vi "DAQNavi Read (Analog Wfm 1Chan NSamp).vi"(8 "error in (no error)":errorcluster, 9 "number of samples per channel to read":u32=1000, 10 "timeout":dbl=10.0, 11 "task in":i32) -> (0 "error out":errorcluster, 1 "markBuf":cluster{"Data Index":i64, "Src Id":i64}[](array[cluster]), 2 "data":waveform(dbl), 3 "task out":i32)   [LabVIEW 2020]
uses:
  DAQNavi_LV.dll
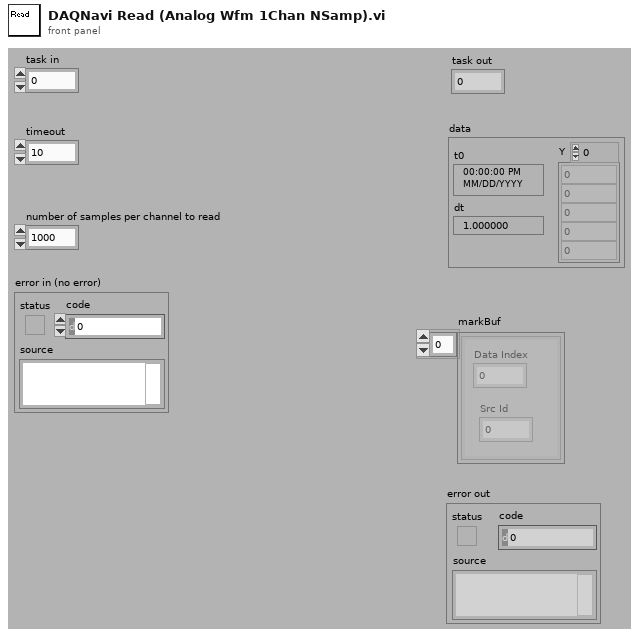
[diagram p1: front panel]
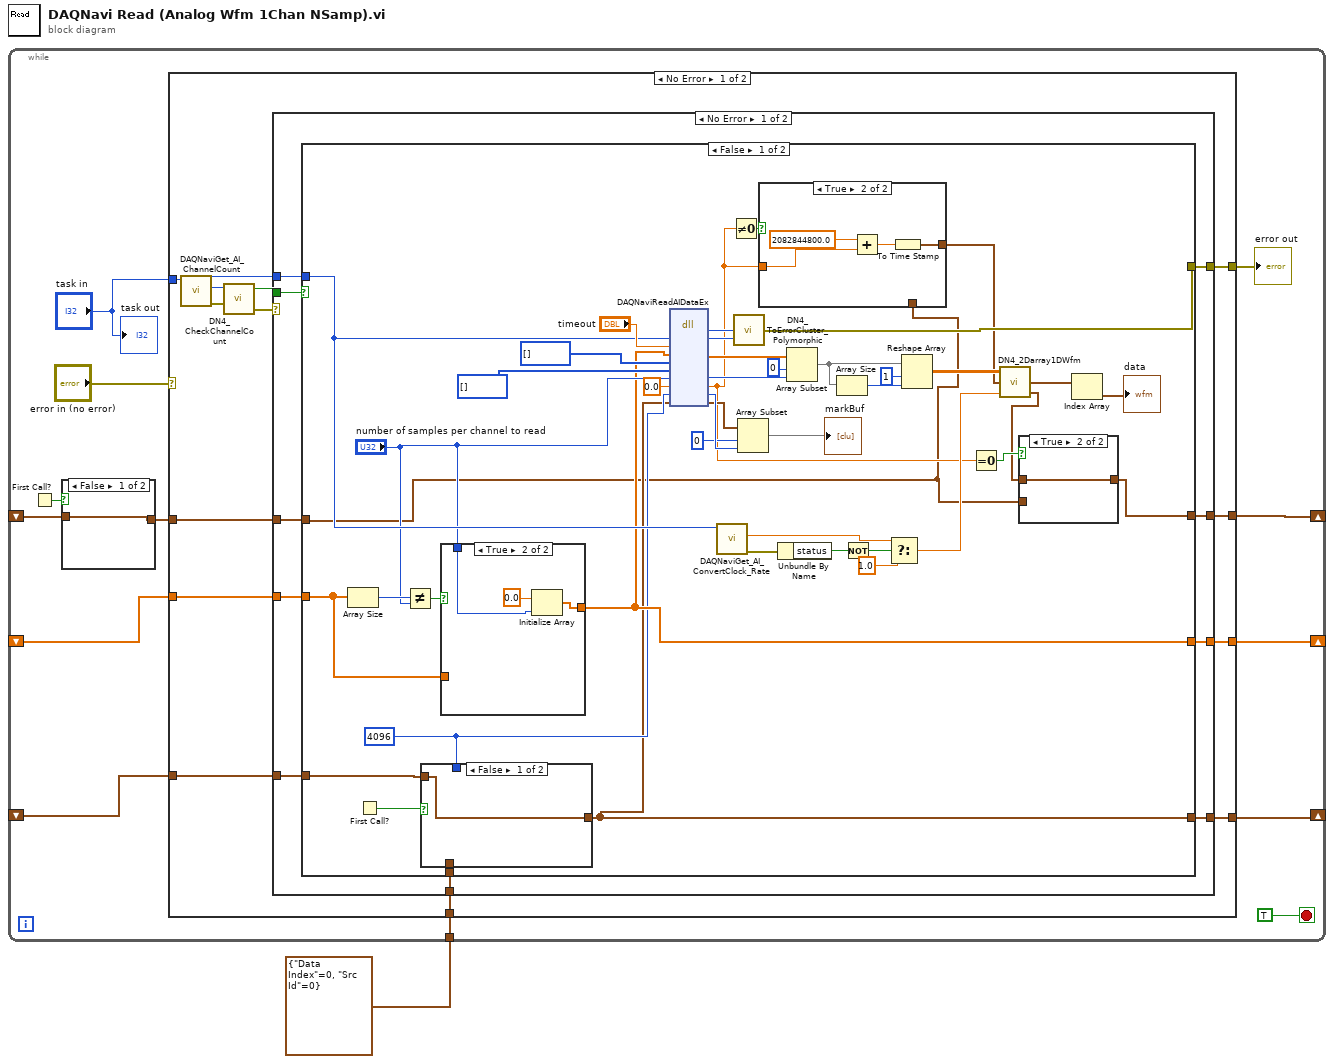
[diagram p0: block diagram]
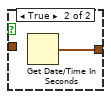
[diagram p2: hidden frame]
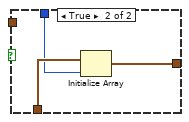
[diagram p3: hidden frame]
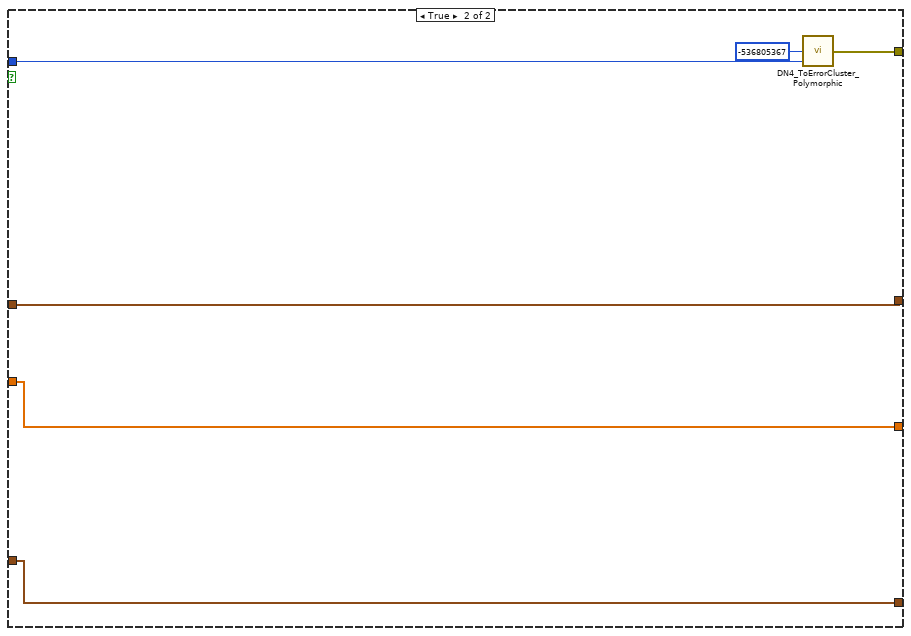
[diagram p7: hidden frame]
diagram:
  n1 = while {
    shift-right: [w8] -> _
    shift-left: _ -> [w7]
    shift-right: [w6] -> _
    shift-left: _ -> [w5]
    tunnel: cluster{"Data Index":i64, "Src Id":i64} {"Data Index"=0, "Src Id"=0} -> [w4]
    shift-right: [w3] -> _
    shift-left: _ -> [w2]
    stop <- TRUE stop-if-true
    n2 = First Call?() -> (First Call?: T/F=w10:bool)
    n3 = case shown="False" w10 {
      tunnel: [w15 w16] -> w9
      tunnel: w7 -> [w15 _]
      frame False {
      }
      frame True {
        n4 = Get Date/Time In Seconds() -> (seconds since 1Jan1904=w16:timestamp)
      }
    }
    n5 = case shown="No Error" "error in (no error)" {
      selector: "error in (no error)" -> [_ w113]
      tunnel: "task in" -> [w30 _]
      tunnel: [w29 w113] -> w13
      tunnel: w9 -> [w23 w112]
      tunnel: [w22 w112] -> w8
      tunnel: [w21 w111] -> w6
      tunnel: w5 -> [w20 w111]
      tunnel: w4 -> [w19 _]
      tunnel: [w18 w110] -> w3
      tunnel: w2 -> [w17 w110]
      frame No Error {
        n6 = call "DAQNaviGet_AI_ChannelCount.vi"("task in"=w30) -> ("error out"=w27:errorcluster, "channel count"=w28:i32, "task out"=w24:i32)  [unwired: 1 in, 7 out]
        n7 = call "DN4_CheckChannelCount.vi"("error out"=w27, "channel count"=w28) -> ("error IO"=w25:errorcluster, "greater than 1?"=w26:bool)  [unwired: 2 out]
        n8 = case shown="No Error" w25 {
          selector: w25 -> [_ w109]
          tunnel: w26 -> [w40 _]
          tunnel: [w39 w109] -> w29
          tunnel: w24 -> [w38 _]
          tunnel: w23 -> [w37 w108]
          tunnel: [w36 w108] -> w22
          tunnel: [w35 w107] -> w21
          tunnel: w20 -> [w34 w107]
          tunnel: w19 -> [w33 _]
          tunnel: [w32 w106] -> w18
          tunnel: w17 -> [w31 w106]
          frame No Error {
            n9 = case shown="False" w40 {
              tunnel: [w80 w104] -> w39
              tunnel: w38 -> [w75 w103]
              tunnel: w37 -> [w42 w102]
              tunnel: [w59 w102] -> w36
              tunnel: [w54 w101] -> w35
              tunnel: w34 -> [w55 w101]
              tunnel: w33 -> [w52 _]
              tunnel: [w49 w100] -> w32
              tunnel: w31 -> [w50 w100]
              frame False {
                w51 = 4096
                n10 = Array Size(array=w55) -> (size(s)=w58:i32)
                n11 = First Call?() -> (First Call?: T/F=w53:bool)
                n12 = Not Equal?(x=w58, y="number of samples per channel to read") -> (x != y?=w56:bool)
                n13 = case shown="False" w53 {
                  tunnel: w52 -> [_ w88]
                  tunnel: w51 -> [_ w87]
                  tunnel: [w85 w86] -> w49
                  tunnel: w50 -> [w85 _]
                  frame False {
                  }
                  frame True {
                    n14 = Initialize Array(w88, w87) -> (w86:cluster{"Data Index":i64, "Src Id":i64}[])
                  }
                }
                n15 = case shown="True" w56 {
                  tunnel: "number of samples per channel to read" -> [_ w91]
                  tunnel: [w89 w90] -> w54
                  tunnel: w55 -> [w89 _]
                  frame False {
                  }
                  frame True {
                    n16 = Initialize Array(0.0 ("element"), w91) -> (w90:dbl[])
                  }
                }
                n17 = dll-call lib="DAQNavi_LV.dll" fn="DAQNaviReadAIDataEx"("taskID"=w75, "timeout"="timeout", "scaledData"=w54, "rawData16"=u16[] [], "rawData32"=u32[] [], "samples"="number of samples per channel to read", "startTime"=0.0, "markCount"=w51, "markBuf"=w49) -> ("return type"=w81:i32, "taskID"=w63:i32, "scaledData"=w79:dbl[], "samples"=w77:u32, "startTime"=w43:dbl, "markCount"=w48:i32, "markBuf"=w46:cluster{"Data Index":i64, "Src Id":i64}[])  [unwired: 4 in, 4 out]
                n18 = call "DAQNaviGet_AI_ConvertClock_Rate.vi"("task in"=w75) -> ("error out"=w74:errorcluster, "rate"=w71:dbl)  [unwired: 1 in, 8 out]
                n19 = Not Equal To 0?(x=w43) -> (x != 0?=w44:bool)
                n20 = call "DN4_ToErrorCluster_Polymorphic.vi"("task id"=w63, "error code"=w81) -> ("error out"=w80:errorcluster)  [unwired: 3 out]
                n21 = Array Subset(array=w46, index=0, length=w48) -> (→"markBuf":cluster{"Data Index":i64, "Src Id":i64}[])
                n22 = case shown="True" w44 {
                  tunnel: w43 -> [_ w99]
                  tunnel: [w95 w97] -> w41
                  tunnel: w42 -> [w95 _]
                  frame False {
                  }
                  frame True {
                    n23 = Add(x=2082844800.0, y=w99) -> (x+y=w96:dbl)
                    n24 = To Time Stamp(1:w96) -> (0:w97:timestamp)
                  }
                }
                n25 = Unbundle By Name(w74) -> ("status"=w73:bool)
                n26 = Array Subset(array=w79, index=0, length=w77) -> (w65:dbl[])
                n27 = Array Size(array=w65) -> (size(s)=w64:i32)
                n28 = Not(x=w73) -> (.not. x?=w72:bool)
                n29 = Select(t=w71, s=w72, f=1.0) -> (s? t:f=w69:dbl)
                n30 = Reshape Array(w65, 1 ("dimension size"), w64) -> (w76:dbl[][])
                n31 = Equal To 0?(x=w43) -> (x = 0?=w61:bool)
                n32 = call "DN4_2Darray1DWfm.vi"("rate"=w69, "StartTime"=w41, "2D Array"=w76) -> ("EndTime"=w60:timestamp, "1D Wfm"=w68:waveform(dbl)[])  [unwired: 1 out]
                n33 = case shown="True" w61 {
                  tunnel: w60 -> [_ w94]
                  tunnel: w42 -> [w93 _]
                  tunnel: [w93 w94] -> w59
                  frame False {
                  }
                  frame True {
                  }
                }
                n34 = Index Array(array=w68) -> (element=→"data":waveform(dbl))  [unwired: 1 in]
              }
              frame True {
                n35 = call "DN4_ToErrorCluster_Polymorphic.vi"("task id"=w103, "error code"=-536805367 ("error code (0)")) -> ("error out"=w104:errorcluster)  [unwired: 3 out]
              }
            }
          }
          frame Error {
          }
        }
      }
      frame Error {
      }
    }
    "error out" <- w13
    "task out" <- "task in"
  }
